vi "FGV_ToTestStandProcessEvent.vi"(7 "Command":T1, 8 "error in":errorcluster) -> (0 "error out":errorcluster, 3 "ToTSProcessEvent":refnum<user-event>)   [LabVIEW 2013]
uses:
  EnumFgvEventCommand.ctl
  ToTestStandProcessEvent.ctl
  ToTestStandProcessEvent - Orders.ctl
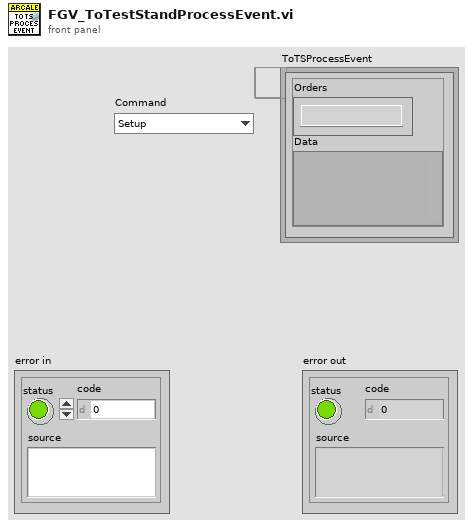
[diagram p1: front panel]
types:
  T1 = typedef "EnumFgvEventCommand.ctl" = enum16{"Setup", "Cleanup", "Get"}
  T2 = typedef "ToTestStandProcessEvent.ctl" = cluster{"Orders":T3, "Data":variant}
  T3 = typedef "ToTestStandProcessEvent - Orders.ctl" = enum16{"Load PMC", "Stop TestSocket Execution", "Change WindowHandle FP"}
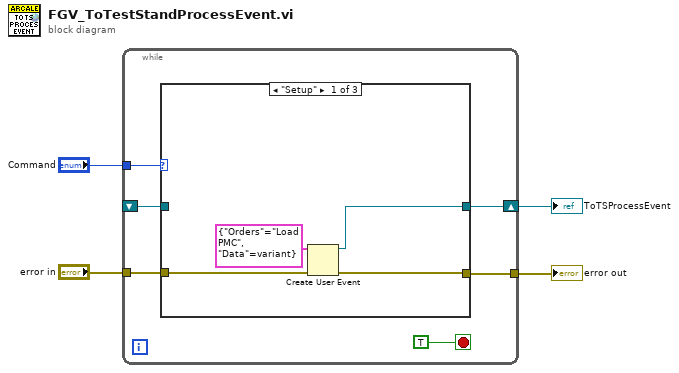
[diagram p0: block diagram]
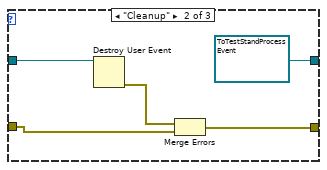
[diagram p2: hidden frame]
diagram:
  n1 = while {
    tunnel: "error in" -> [w8]
    tunnel: "Command" -> [w9]
    tunnel: [w7] -> w2
    shift-right: [w6] -> w1
    shift-left: _ -> [w5]
    stop <- TRUE stop-if-true
    n2 = case shown="\"Setup\"" w9 {
      tunnel: w8 -> [w14 w18 w20]
      tunnel: [w13 w16 w20] -> w7
      tunnel: [w12 refnum<user-event> refnum ("user event out") w21] -> w6
      tunnel: w5 -> [_ w19 w21]
      frame "Setup" {
        n3 = Create User Event(user event datatype=T2 {"Orders"=enum."Load PMC", "Data"=variant} ("ToTestStandProcessEvent"), error in=w14) -> (user event=w12:refnum<user-event>, error out=w13:errorcluster)
      }
      frame "Cleanup" {
        n4 = Destroy User Event(user event=w19) -> (error out=w17:errorcluster)  [unwired: 1 in]
        n5 = Merge Errors(w17, w18) -> (w16:errorcluster)
      }
      frame "Get" {
      }
    }
  }
  "error out" <- w2
  "ToTSProcessEvent" <- w1
